vi "Update Channel Data.vi"(8 "error in (no error)":errorcluster, 10 "ChannelData":refnum<class "ChannelData.lvclass">, 11 "Channel in":refnum<class "Channel.lvclass">) -> (0 "error out":errorcluster, 3 "Channel out":refnum<class "Channel.lvclass">)   [LabVIEW 2015, in "Channel.lvlib" / "Channel.lvclass"]
uses:
  Channel.lvclass
  ChannelData.lvclass
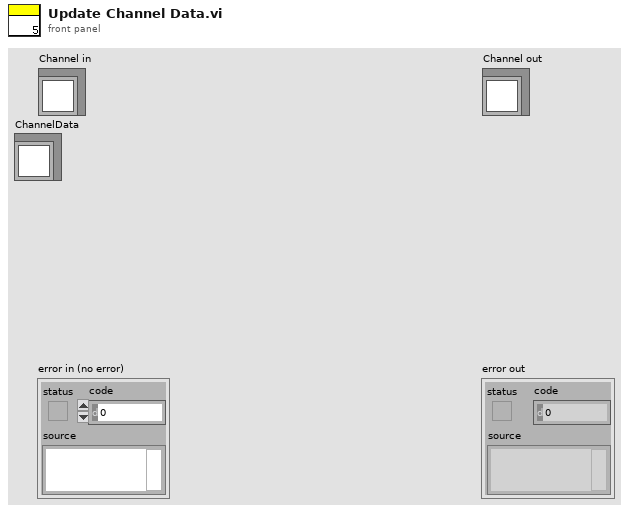
[diagram p1: front panel]
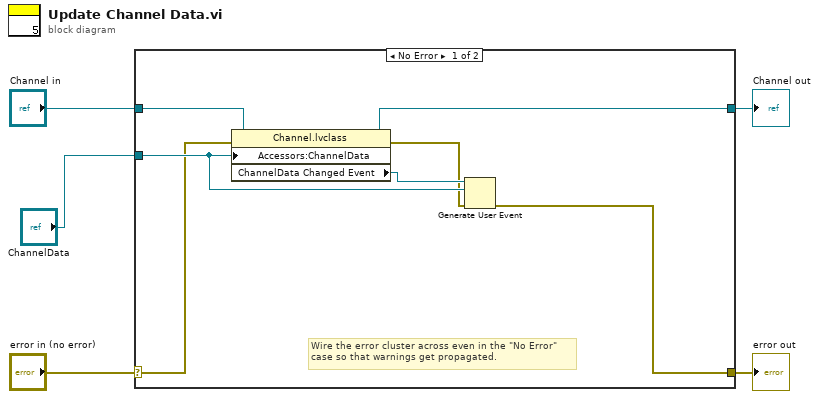
[diagram p0: block diagram]
diagram:
  n1 = case shown="No Error" "error in (no error)" {
    selector: "error in (no error)" -> [w8 w14]
    tunnel: [w6 w14] -> w4
    tunnel: [w11 w13] -> w2
    tunnel: "Channel in" -> [w12 w13]
    tunnel: "ChannelData" -> [w10 _]
    frame No Error {
      # "Wire the error cluster across even in the \"No Error\"\ncase so that warnings get propagated."
      n2 = property class="Channel.lvclass"(reference=w12, error in=w8, "Accessors:ChannelData"=w10) -> (reference out=w11:refnum<class "Channel.lvclass">, error out=w7:errorcluster, "ChannelData Changed Event"=w9:refnum<user-event>)
      n3 = Generate User Event(user event=w9, event data cluster=w10, error in=w7) -> (error out=w6:errorcluster)  [unwired: 1 in, 1 out]
    }
    frame Error {
    }
  }
  "error out" <- w4
  "Channel out" <- w2
